vi "RT Driver VI.vi"(6 "Device Clock":string, 9 "Device Inputs FIFO":refnum<k33>, 10 "Device Outputs FIFO":refnum<k33>, 11 "Device Reference":T1 format="%.0x") -> ()   [LabVIEW 2020, in "gRPC Data Server Engine.lvlib"]
uses:
  <vilib>/NI VeriStand/Custom Device API/Custom Device Item Ref.ctl
  <vilib>/NI VeriStand/Custom Device API/Message Response (String).ctl
  <vilib>/NI VeriStand/Custom Device API/Message Response (Byte Array).ctl
  gRPC Data Server Engine.lvlib
  <vilib>/NI VeriStand/Custom Device Tools/Custom Device Utility Library/Custom Device Utility Library.lvlib
  <vilib>/NI VeriStand/Custom Device API/Custom Device API.lvlib
  Shared/Constants.vi
  Shared/gRPC Data Server Shared.lvlib
  Shared/Compiled.Settings.ctl
  <vilib>/gRPC/LabVIEW gRPC Servicer/Servicer/Servicer.lvclass
  editor-plugin-source/labview-source/veristand-grpc_server/Veristandgrpc_server.lvlib
  editor-plugin-source/labview-source/veristand-grpc_server/RPC Service/veristand/veristand-grpc.lvclass
  editor-plugin-source/labview-source/veristand-grpc_server/Data/Data Server.lvclass
  <vilib>/NI VeriStand/Custom Device API/Get Item Property (Variant).vi
panel:
  out "Listening Port":i32
  in  "Initialization Status Notifier":refnum<notifier>
  in  "Status Notifier":refnum<notifier>
  # "Custom Device Template\nv1.0"
  # "Use this template as a starting point for creating a custom device code module. The input controls shown here are specially named controls that the system will use to provide the device loop with data. The controls are not required for the device loop to run. For instance, if the device doesn't produce any output data, then you don't need the Device Outputs FIFO control. If you do use these controls, however, they need to have these exact names to be functional."
  # "The optional status notifier element is used to notify the RT engine of the last state of the custom device, and to indicate the device has completed execution. If this control is not used, a default No Error value is returned to the system when the device finishes execution.\n\nNote: This error state is not checked until the system shuts down. Use an output status channel to send more immediate status values to the system."
  # "This optional input can be used to send the VeriStand Engine the final status of the custom device initalization process. If this control exists on the custom device front panel, the VeriStand Engine will wait for a status update before starting up. If the custom device reports an error, that will abort the execution of the current configuration in the VeriStand Engine.\n\nThis control can be deleted if the custom device does not need to send the initialization status update."
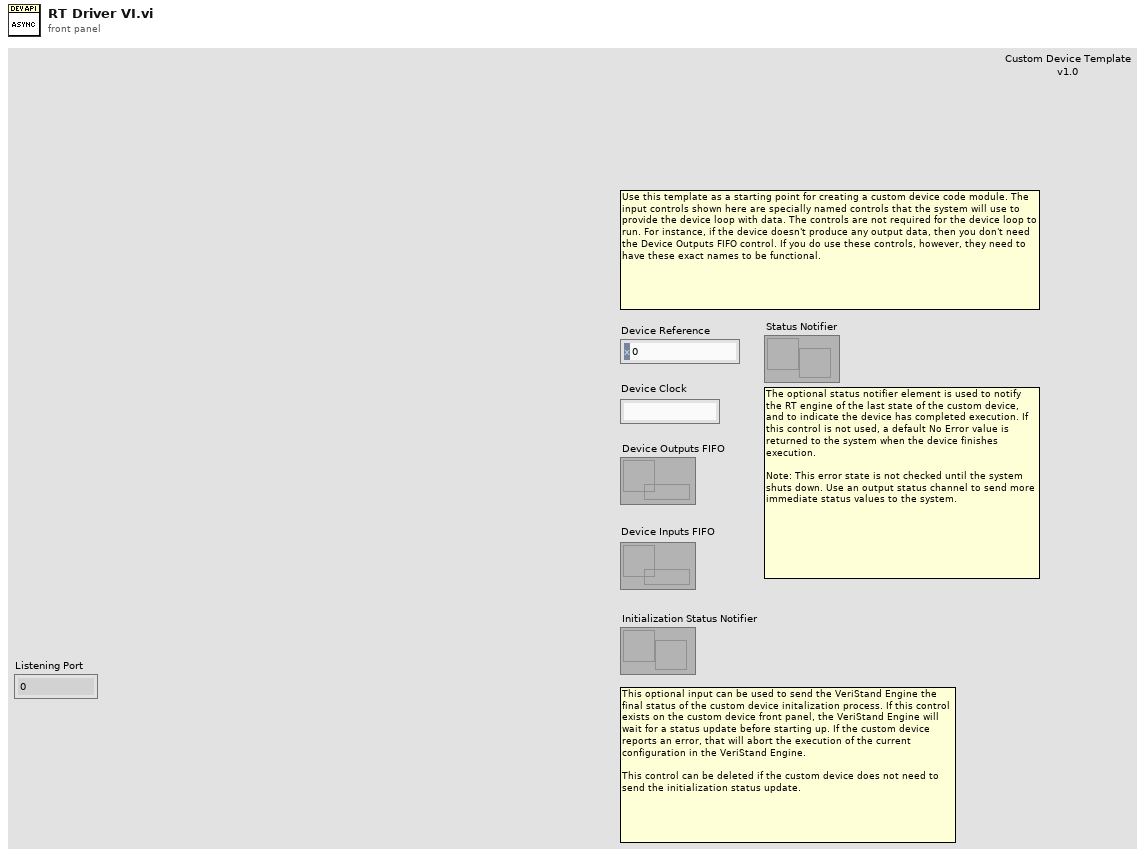
[diagram p1: front panel]
types:
  T1 = typedef "Custom Device API.lvlib/Custom Device Item Ref.ctl" = u64
  T2 = typedef "gRPC Data Server Shared.lvlib/Compiled.Settings.ctl" = cluster{"Name":string, "Server Address":string, "Async?":bool, "Key File":path, "Cert File":path, "Channel Name":string[], "Initial Value":string[]}
  T3 = typedef "Custom Device API.lvlib/Custom Device Engine Event Ref.ctl" = refnum<event-registration>
  T4 = typedef "grpc-lvsupport-release.lvlib/grpcId.ctl" = u64
  T5 = typedef "Custom Device API.lvlib/Message Response (String).ctl" = cluster{"Response":string, "Error":errorcluster}
  T6 = typedef "Custom Device API.lvlib/Message Response (Byte Array).ctl" = cluster{"Response":u8[], "Error":errorcluster}
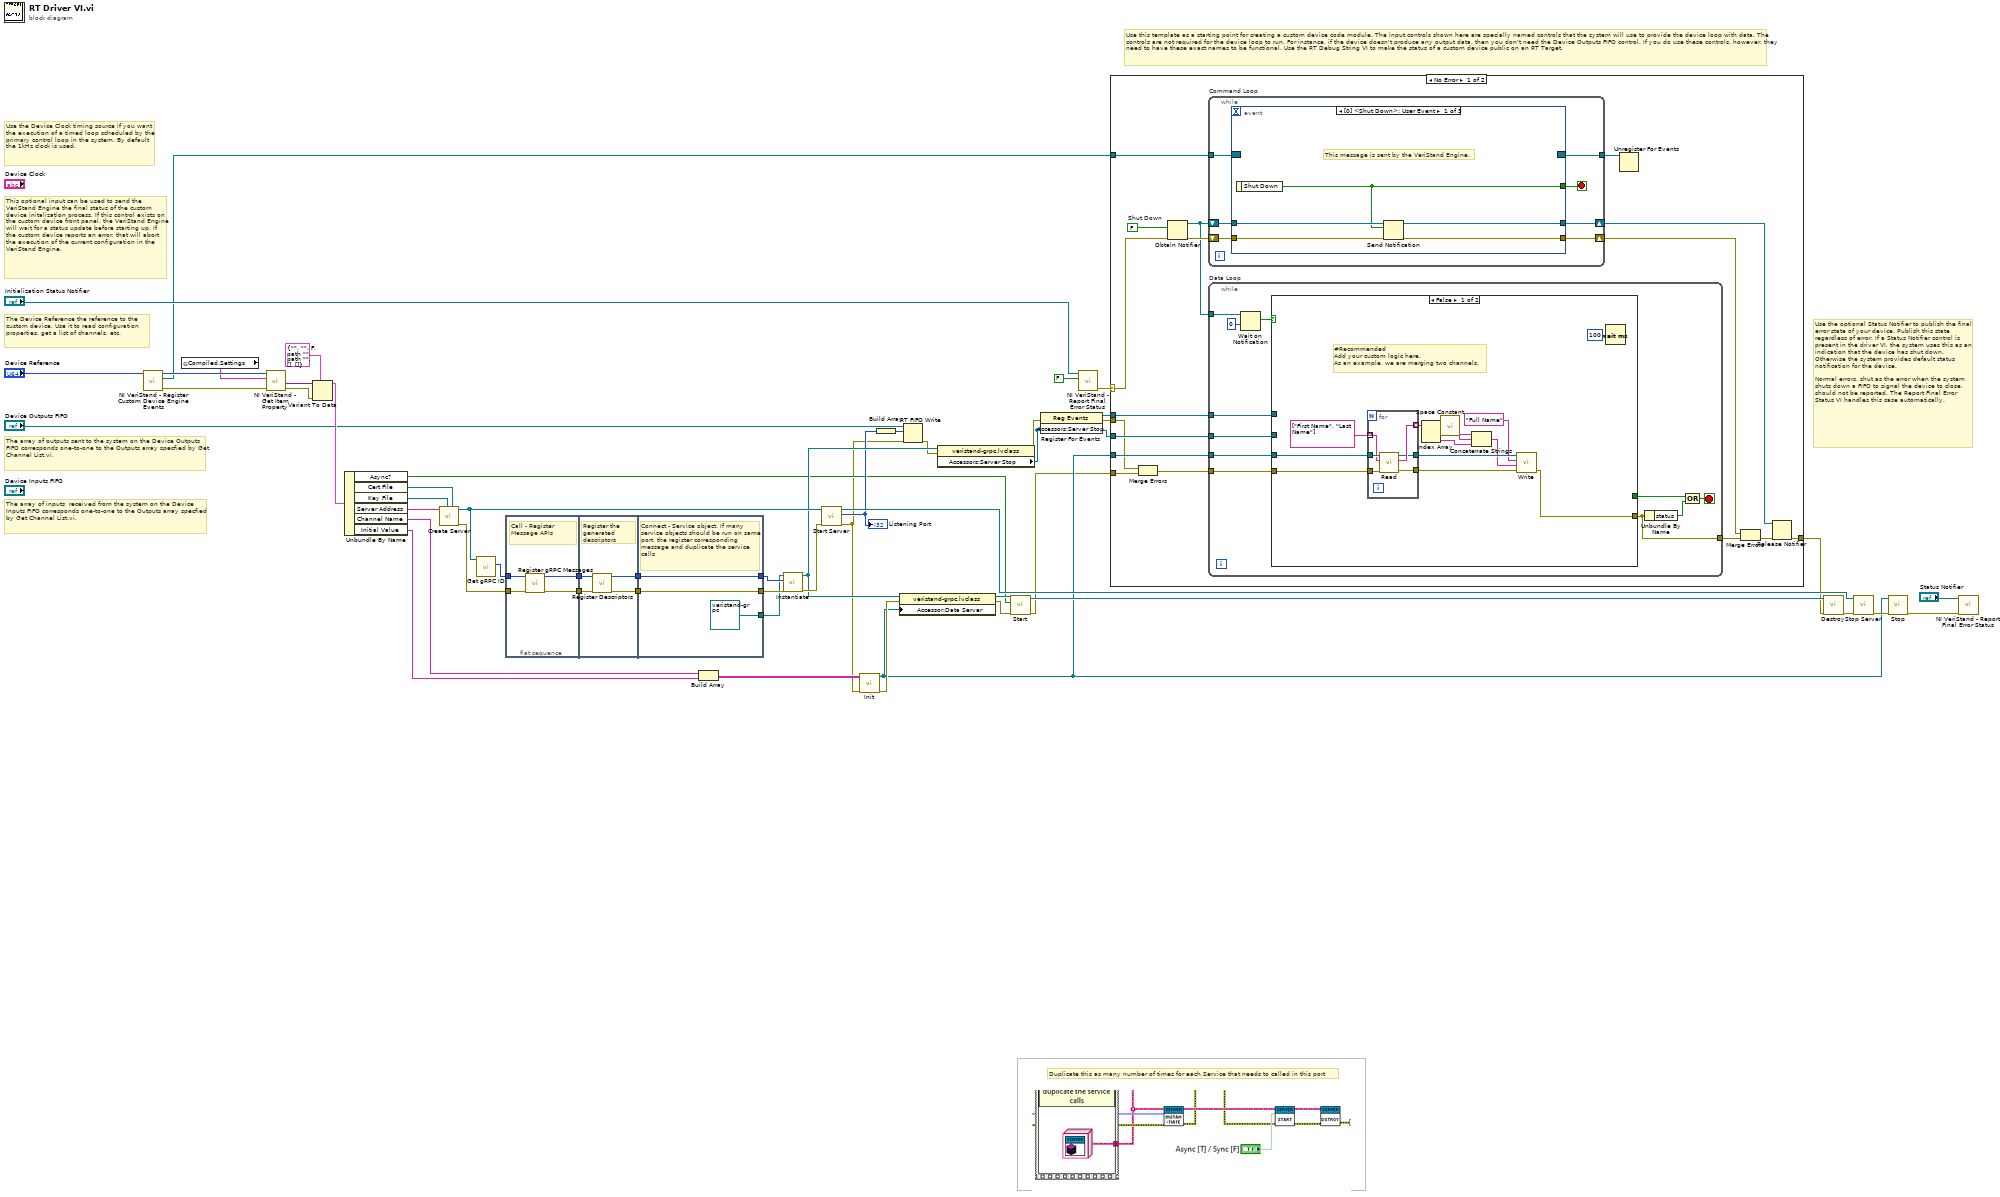
[diagram p0: block diagram]
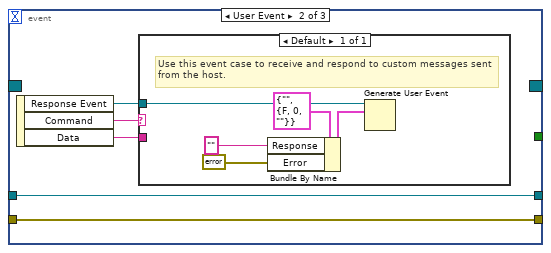
[diagram p2: hidden frame]
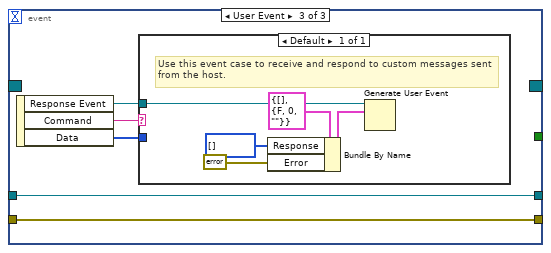
[diagram p3: hidden frame]
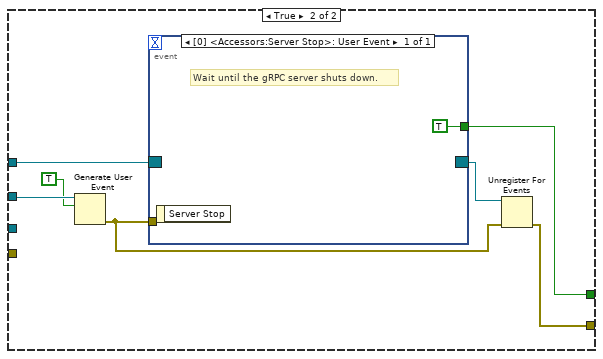
[diagram p4: hidden frame]
diagram:
  # "Duplicate this as many number of times for each Service that needs to called in this port"
  # "This optional input can be used to send the VeriStand Engine the final status of the custom device initalization process. If this control exists on the custom device front panel, the VeriStand Engine will wait for a status update before starting up. If the custom device reports an error, that will abort the execution of the current configuration in the VeriStand Engine."
  # "The array of inputs  received from the system on the Device Inputs FIFO corresponds one-to-one to the Outputs array specfied by Get Channel List.vi."
  # "Use the optional Status Notifier to publish the final error state of your device. Publish this state regardless of error. If a Status Notifier control is present in the driver VI, the system uses this as an indication that the device has shut down. Otherwise the system provides default status notification for the device.\n\nNormal errors, shut as the error when the system shuts down a FIFO to signal the device to close, should not be reported. The Report Final Error Status VI handles this case automatically."
  # "The array of outputs sent to the system on the Device Outputs FIFO corresponds one-to-one to the Outputs array specfied by Get Channel List.vi."
  # "The Device Reference the reference to the custom device. Use it to read configuration properties, get a list of channels, etc."
  # "Use the Device Clock timing source if you want the execution of a timed loop scheduled by the primary control loop in the system. By default the 1kHz clock is used."
  # "Use this template as a starting point for creating a custom device code module. The input controls shown here are specially named controls that the system will use to provide the device loop with data. The controls are not required for the device loop to run. For instance, if the device doesn't produce any output data, then you don't need the Device Outputs FIFO control. If you do use these controls, however, they need to have these exact names to be functional. Use the RT Debug String VI to make the status of a custom device public on an RT Target."
  n1 = call <vilib>:"NI VeriStand - Register Custom Device Engine Events.vi"("Device Ref in"="Device Reference") -> ("error out"=w46:errorcluster, "Custom Device Engine Event Ref"=w10:T3, "Device Ref out"=w47:T1)  [unwired: 8 in]
  n2 = global read "Constants.vi" "Compiled.Settings"() -> (w45:string)
  n3 = call-poly <vilib>:"NI VeriStand - Get Item Property.vi"("error in (no error)"=w46, "Property Name"=w45, "Item Ref in"=w47) -> ("error out"=w44:errorcluster, "Value"=w43:variant)  [unwired: 5 in, 2 out]
  n4 = Variant To Data(error in=w44, type=T2 {"Name"="", "Server Address"="", "Async?"=FALSE, "Key File"=path "", "Cert File"=path "", "Channel Name"=[], "Initial Value"=[]} ("Compiled.Settings"), Variant=w43) -> (data=w21:T2)  [unwired: 1 out]
  n5 = Unbundle By Name(w21) -> ("Async?"=w11:bool, "Cert File"=w18:path, "Key File"=w19:path, "Server Address"=w20:string, "Channel Name"=w16:string[], "Initial Value"=w15:string[])
  n6 = call <vilib>:"Create Server.vi"("Server Key File (.key)"=w18, "Server Certificate File (.crt)"=w19, "Server Address"=w20) -> ("error out"=w31:errorcluster, "gRPC Server out"=w36:refnum<class "Servicer.lvclass">)  [unwired: 7 in]
  n7 = call <vilib>:"Get gRPC ID.vi"("OOP Server in"=w36) -> ("gRPC ID"=w32:T4)  [unwired: 9 in, 1 out]
  n8 = flat-sequence {
    tunnel: w32 -> [w54]
    tunnel: w31 -> [w56]
    tunnel: [w55] -> w41
    tunnel: [w53] -> w40
    tunnel: w41 -> [w59]
    tunnel: w40 -> [w60]
    tunnel: [w57] -> w39
    tunnel: [w58] -> w38
    tunnel: [w62] -> w29
    tunnel: [w63] -> w30
    tunnel: w39 -> [w63]
    tunnel: w38 -> [w62]
    tunnel: [refnum<class "veristand-grpc.lvclass"> refnum ("veristand-grpc_server.lvlib:veristand.lvclass")] -> w27
    frame #0 {
      # "Call - Register Message APIs"
      n9 = call "Register gRPC Messages.vi"("error in (no error)"=w56, "gRPC ID"=w54) -> ("error out"=w55:errorcluster, "gRPC ID Out"=w53:T4)  [unwired: 8 in]
    }
    frame #1 {
      # "Register the generated descriptors"
      n10 = call "Register Descriptors.vi"("error in (no error)"=w59, "gRPC ID"=w60) -> ("error out"=w57:errorcluster, "gRPC ID Out"=w58:T4)  [unwired: 8 in]
    }
    frame #2 {
      # "Connect - Service object. If many service objects should be run on same port, the register corresponding message and duplicate the service calls"
    }
  }
  n11 = Build Array(w16, w15) -> (w14:string[][])
  n12 = call-dynamic "Instantiate.vi"("error in"=w30, "gRPCid"=w29, "iService"=w27) -> ("error out"=w34:errorcluster, "iService"=w26:refnum<class "veristand-grpc.lvclass">)  [unwired: 7 in]
  n13 = call <vilib>:"Start Server.vi"("error in"=w34, "gRPC Server in"=w36) -> ("error out"=w8:errorcluster, "Listening Port"=w13:i32, "gRPC Server out"=w37:refnum<class "Servicer.lvclass">)  [unwired: 7 in]
  "Listening Port" <- w13
  n14 = call "Init.vi"("error in (no error)"=w8, "Initial Data"=w14) -> ("error out"=w22:errorcluster, "DVR out"=w3:refnum<class "Data Server.lvclass">)  [unwired: 8 in]
  n15 = Build Array(w13) -> (w12:i32[])
  n16 = property class="veristand-grpc.lvclass"(reference=w26, error in=w22, "Accessor:Data Server"=w3) -> (reference out=w25:refnum<class "veristand-grpc.lvclass">, error out=w24:errorcluster)
  n17 = RT FIFO Write(0:"Device Outputs FIFO", 1:w12, 3:w8) -> (11:w7:errorcluster)  [unwired: 1 in, 4 out]
  n18 = property class="veristand-grpc.lvclass"(reference=w26, error in=w7) -> (error out=w35:errorcluster, "Accessors:Server Stop"=w9:refnum<user-event>)  [unwired: 1 out]
  n19 = call-dynamic "Start.vi"("error in"=w24, "ASync [T]"=w11, "iService in"=w25) -> ("error out"=w1:errorcluster, "iService out"=w28:refnum<class "veristand-grpc.lvclass">)  [unwired: 7 in]
  n20 = register-events(error in=w35, w9) -> (reference out=w6:refnum<event-registration>, error out=w2:errorcluster)  [unwired: 1 in]
  n21 = call <vilib>:"NI VeriStand - Report Final Error Status.vi"("Filter FIFO & Shutdown Errors (T)"=FALSE ("Filter FIFO Errors (T)"), "Status Notifier"="Initialization Status Notifier") -> ("error out"=w49:errorcluster)  [unwired: 1 in, 8 out]
  n22 = case shown="No Error" w49 {
    selector: w49 -> [w73 w151]
    tunnel: w10 -> [w79 _]
    tunnel: [w77 w151] -> w5
    tunnel: w9 -> [w70 _]
    tunnel: w6 -> [w69 _]
    tunnel: w3 -> [w68 _]
    tunnel: w2 -> [w67 _]
    tunnel: w1 -> [w66 _]
    frame No Error {
      w78 = FALSE  # Shut Down
      n23 = Merge Errors(w67, w66) -> (w65:errorcluster)
      n24 = Obtain Notifier(notification data type=w78, error in (no error)=w73) -> (notifier out=w75:refnum<notifier>, error out=w80:errorcluster)  [unwired: 2 in, 1 out]
      n25 = while "Command Loop" {
        tunnel: w79 -> [w87]
        tunnel: [w86] -> w76
        shift-right: [w83] -> w74
        shift-left: w75 -> [w84]
        shift-right: [w81] -> w71
        shift-left: w80 -> [w82]
        stop <- w85 stop-if-true
        n26 = event shown="[0] <Shut Down>: User Event" {
          selector: w87 -> [_ _ _]
          dyn-events: [_ _ _] -> w86
          timeout: _ -> [_ _ _]
          tunnel: [w90 _ _] -> w85
          tunnel: w84 -> [w91 w95 w105]
          tunnel: [w92 w95 w105] -> w83
          tunnel: w82 -> [w89 w93 w103]
          tunnel: [w88 w93 w103] -> w81
          event User Event {
            # "This message is sent by the VeriStand Engine."
            n27 = event-data() -> ("Shut Down"=w90:bool)  [unwired: 1 in]
            n28 = Send Notification(notification=w90, notifier=w91, error in (no error)=w89) -> (notifier out=w92:refnum<notifier>, error out=w88:errorcluster)
          }
          event User Event {
            n29 = event-data() -> ("Response Event"=w94:refnum<user-event>, "Command"=w97:string, "Data"=w96:string)  [unwired: 1 in]
            n30 = case shown="Default" w97 {
              tunnel: w96 -> [_]
              tunnel: w94 -> [w102]
              frame Default {
                # "Use this event case to receive and respond to custom messages sent from the host."
                n31 = Bundle By Name(cluster=T5 {"Response"="", "Error"={"status"=FALSE, "code"=0, "source"=""}} ("event data"), "Response"="", "Error"=errorcluster {"status"=FALSE, "code"=0, "source"=""}) -> (w100:T5)
                n32 = Generate User Event(user event=w102, event data cluster=w100) -> ()  [unwired: 2 in, 2 out]
              }
            }
          }
          event User Event {
            n33 = event-data() -> ("Response Event"=w104:refnum<user-event>, "Command"=w107:string, "Data"=w106:u8[])  [unwired: 1 in]
            n34 = case shown="Default" w107 {
              tunnel: w106 -> [_]
              tunnel: w104 -> [w112]
              frame Default {
                # "Use this event case to receive and respond to custom messages sent from the host."
                n35 = Bundle By Name(cluster=T6 {"Response"=[], "Error"={"status"=FALSE, "code"=0, "source"=""}} ("event data"), "Response"=u8[] [], "Error"=errorcluster {"status"=FALSE, "code"=0, "source"=""}) -> (w109:T6)
                n36 = Generate User Event(user event=w112, event data cluster=w109) -> ()  [unwired: 2 in, 2 out]
              }
            }
          }
        }
      }
      n37 = while "Data Loop" {
        tunnel: w75 -> [w122]
        tunnel: w70 -> [w118]
        tunnel: w69 -> [w117]
        tunnel: w68 -> [w115]
        tunnel: w65 -> [w114]
        tunnel: [w113] -> w64
        stop <- w119 stop-if-true
        n38 = Wait on Notification(notifier=w122, timeout in ms (-1)=0) -> (notification=w121:bool)  [unwired: 2 in, 3 out]
        n39 = case shown="False" w121 {
          tunnel: [_ w146] -> w120
          tunnel: w118 -> [_ w148]
          tunnel: w117 -> [_ w149]
          tunnel: w115 -> [w135 _]
          tunnel: w114 -> [w134 _]
          tunnel: [w124 w143] -> w113
          frame False {
            # "#Recommended\nAdd your custom logic here.\nAs an example, we are merging two channels."
            n40 = for {
              tunnel: w135 -> [w142]
              tunnel: w134 -> [w141]
              tunnel: string[] ["First Name", "Last Name"] -> [w140] mode=indexing
              tunnel: [w139] -> w132 mode=indexing
              tunnel: [w138] -> w128
              tunnel: [w137] -> w127
              n41 = call "Read.vi"("error in (no error)"=w141, "Channel Name"=w140, "Data in"=w142) -> ("error out"=w137:errorcluster, "Data"=w139:string, "Data out"=w138:refnum<class "Data Server.lvclass">)  [unwired: 5 in, 1 out]
            }
            n42 = Index Array(array=w132) -> (element #1=w131:string, element #2=w129:string)  [unwired: 2 in]
            n43 = call <vilib>:"Space Constant.vi"() -> ("String"=w130:string)
            n44 = Concatenate Strings(w131, w130, w129) -> (w126:string)
            n45 = call "Write.vi"("error in (no error)"=w127, "New Data"=w126, "Channel Name"="Full Name", "Data in"=w128) -> ("error out"=w124:errorcluster)  [unwired: 5 in, 2 out]
            n46 = Wait (ms)(milliseconds to wait=u32 100) -> ()  [unwired: 1 out]
          }
          frame True {
            n47 = Generate User Event(user event=w148, event data cluster=TRUE ("event data")) -> (error out=w144:errorcluster)  [unwired: 2 in, 1 out]
            n48 = event shown="[0] <Accessors:Server Stop>: User Event" {
              selector: w149 -> [_]
              dyn-events: [_] -> w145
              timeout: _ -> [_]
              tunnel: [TRUE] -> w146
              tunnel: w144 -> [_]
              event User Event {
                # "Wait until the gRPC server shuts down."
                n49 = event-data() -> ()  [unwired: 1 in, 1 out]
              }
            }
            n50 = Unregister For Events(event registration refnum=w145, error in=w144) -> (error out=w143:errorcluster)
          }
        }
        n51 = Unbundle By Name(w113) -> ("status"=w116:bool)
        n52 = Compound Arithmetic op=OR(w120, w116) -> (w119:bool)
      }
      n53 = Unregister For Events(event registration refnum=w76) -> ()  [unwired: 1 in, 1 out]
      n54 = Merge Errors(w71, w64) -> (w72:errorcluster)
      n55 = Release Notifier(notifier=w74, error in (no error)=w72) -> (error out=w77:errorcluster)  [unwired: 1 in, 2 out]
    }
    frame Error {
    }
  }
  n56 = call-dynamic "Destroy.vi"("error in (no error)"=w5, "SignalGeneratorService in"=w28) -> ("error out"=w33:errorcluster)  [unwired: 8 in, 1 out]
  n57 = call <vilib>:"Stop Server.vi"("error in"=w33, "gRPC Server in"=w37) -> ("error out"=w23:errorcluster)  [unwired: 9 in]
  n58 = call "Stop.vi"("error in (no error)"=w23, "DVR in"=w3) -> ("error out"=w4:errorcluster)  [unwired: 9 in]
  n59 = call <vilib>:"NI VeriStand - Report Final Error Status.vi"("error in (no error)"=w4, "Status Notifier"="Status Notifier") -> ()  [unwired: 1 in, 9 out]
